vi "FGPAGlobals.vi"() -> ()   [LabVIEW 2018]
panel:
  out "pos/cur 2 internal mode":bool
  out "pos/cur internal mode":bool
  out "TrigAI 2":bool
  out "Position Loop Current 2":i16
  out "Position Loop Current 1":i16
  out "TrigAI":bool
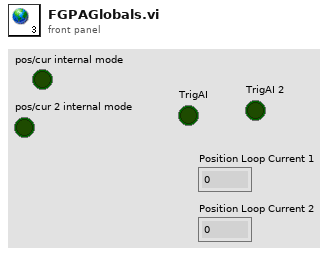
[diagram p1: front panel]
diagram:
